vi "H5Pset_fill_value.vi"(4 "Data Element":variant, 5 "HDF5 Type Ref (match data)":T1, 6 "error in (no error)":errorcluster, 9 "HDF5 Property Ref":T1) -> (0 "error out":errorcluster, 3 "HDF5 Ref out":T1)   [LabVIEW 2017]
doc: "Sets the fill value for a dataset."
uses:
  <vilib>/UPVI/lvhdf5/library.llb/HDF5 Ref.ctl
  <vilib>/UPVI/lvhdf5/identifier.llb/H5Iget_type.vi
  <vilib>/UPVI/lvhdf5/h5helper.dll
panel:
  # "LVHDF5 Toolkit\nCopyright (c) 2005-2013 by Jason D. Sommerville\nCopyright (c) 2014 by UPVI, LLC.\n\nThis use and distribution of this file is governed by the terms found in \nLICENSE.txt distributed with this toolkit and installed at\n <user.lib>\\_lvhdf5\\LICENSE.txt"
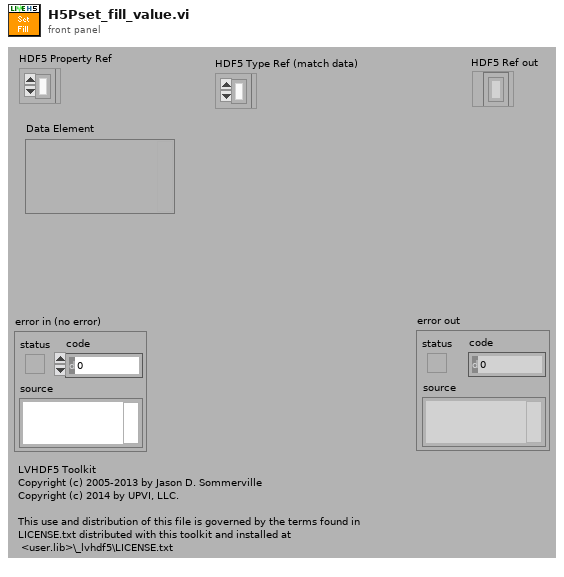
[diagram p1: front panel]
types:
  T1 = typedef "HDF5 Ref.ctl" = refnum<k1>
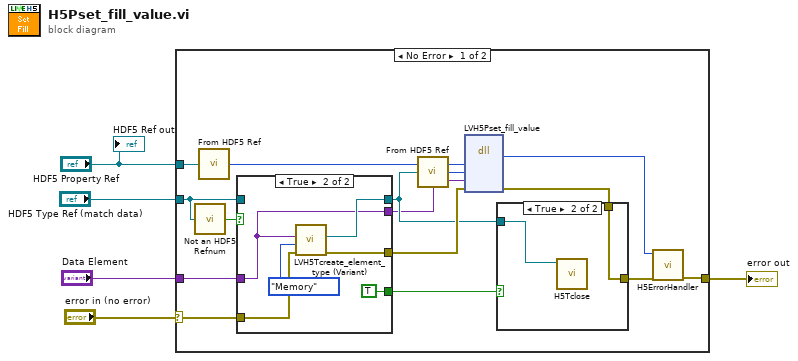
[diagram p0: block diagram]
diagram:
  n1 = case shown="No Error" "error in (no error)" {
    selector: "error in (no error)" -> [w15 w33]
    tunnel: [w7 w33] -> w4
    tunnel: "HDF5 Property Ref" -> [w20 _]
    tunnel: "Data Element" -> [w13 _]
    tunnel: "HDF5 Type Ref (match data)" -> [w16 _]
    frame No Error {
      n2 = call <vilib>:"Not an HDF5 Refnum.vi"("HDF5 Ref"=w16) -> ("Not an HDF5 Refnum"=w17:bool)
      n3 = call <vilib>:"From HDF5 Ref.vi"("HDF5 Ref"=w20) -> ("I32"=w19:i32)
      n4 = case shown="True" w17 {
        tunnel: w16 -> [w26 _]
        tunnel: [w26 w29] -> w11
        tunnel: w15 -> [w25 w32]
        tunnel: [w25 w31] -> w14
        tunnel: w13 -> [w24 w27]
        tunnel: [_ TRUE] -> w10
        tunnel: [w24 w27] -> w9
        frame False {
        }
        frame True {
          n5 = call <vilib>:"LVH5Tcreate_element_type (Variant).vi"("error in (no error)"=w32, "Type"=enum16{"File", "Memory"}."Memory", "Data"=w27) -> ("error out"=w31:errorcluster, "HDF5 Type Ref"=w29:T1)  [unwired: 4 in, 3 out]
        }
      }
      n6 = call <vilib>:"From HDF5 Ref.vi"("HDF5 Ref"=w11) -> ("I32"=w18:i32)
      n7 = dll-call lib="C:/Program Files/National Instruments/LabVIEW 2017/vi.lib/UPVI/lvhdf5/h5helper.dll" fn="LVH5Pset_fill_value"("plist_id"=w19, "type_id"=w18, "plvvar"=w9, "error"=w14) -> ("return type"=w6:i32, "error"=w12:errorcluster)  [unwired: 6 in, 2 out]
      n8 = case shown="True" w10 {
        tunnel: w11 -> [_ w23]
        tunnel: w12 -> [w21 w22]
        tunnel: [w21 w22] -> w8
        frame False {
        }
        frame True {
          n9 = call <vilib>:"H5Tclose.vi"("HDF5 Datatype Ref"=w23) -> ()  [unwired: 8 in, 1 out]
        }
      }
      n10 = call <vilib>:"H5ErrorHandler.vi"("error in (no error)"=w8, "herr_t"=w6) -> ("error out"=w7:errorcluster)  [unwired: 3 in, 4 out]
    }
    frame Error {
    }
  }
  "error out" <- w4
  "HDF5 Ref out" <- "HDF5 Property Ref"
